vi "View.vi"(8 "error in (no error)":errorcluster, 11 "Worker In":refnum<class "Worker.lvclass">) -> (0 "error out":errorcluster)   [LabVIEW 2020, in "Worker.lvclass"]
doc: "This VI implements the main UI of the process. A reference to this VI should be set using the Set View VI Reference.vi method when the VI is started."
uses:
  Worker.lvclass
  C:/Program Files (x86)/National Instruments/LabVIEW 2020/vi.lib/Astemes/Triarc Framework/Process/Process.lvclass
  C:/Program Files (x86)/National Instruments/LabVIEW 2020/vi.lib/Astemes/Triarc Framework/View/View.lvclass
  <vilib>/Astemes/Triarc Framework/View/View.lvclass/View.ctl
  <vilib>/Astemes/Triarc Framework/View/View.lvclass
  <vilib>/Astemes/Triarc Framework/Process/Process.lvclass
panel:
  out "Name":string
  out "Worker Type":string="Barista"
  out "Orders Filled This Shift":u32
  out "Status":string
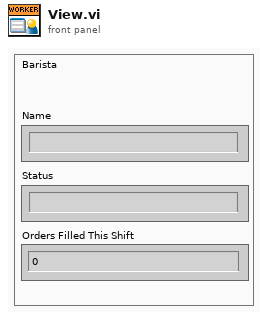
[diagram p1: front panel]
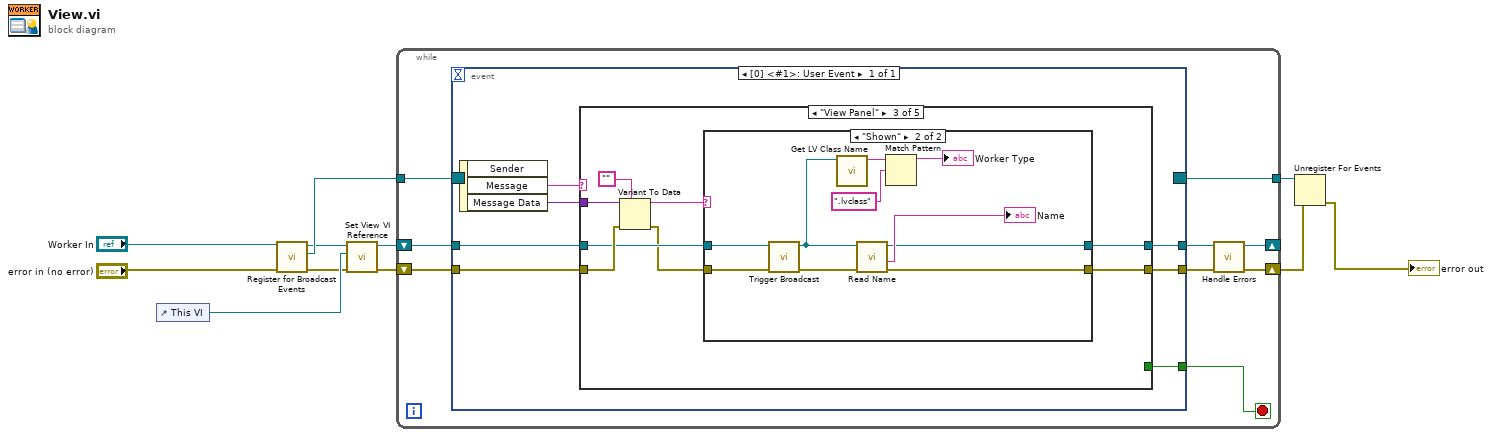
[diagram p0: block diagram]
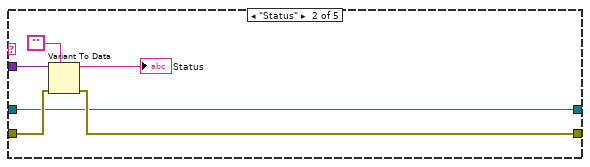
[diagram p3: hidden frame]
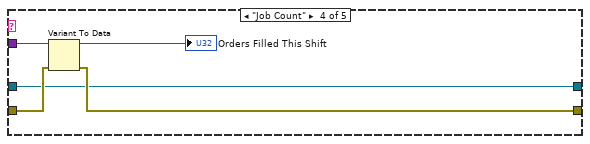
[diagram p5: hidden frame]
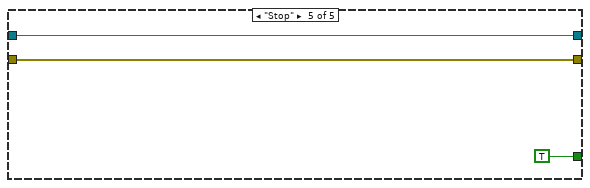
[diagram p6: hidden frame]
diagram:
  n1 = control-ref of="This VI"() -> (w10:refnum<vi>)
  n2 = call <vilib>:"Register for Broadcast Events.vi"("error in (no error)"="error in (no error)", "Process In"="Worker In") -> ("error out"=w8:errorcluster, "Event Registration Refnum Out"=w9:refnum<event-registration>, "Process Out"=w7:refnum<class "Worker.lvclass">)  [unwired: 7 in]
  n3 = call <vilib>:"Set View VI Reference.vi"("error in (no error)"=w8, "View VI Reference"=w10, "View In"=w7) -> ("error out"=w6:errorcluster, "View Out"=w5:refnum<class "Worker.lvclass">)  [unwired: 7 in]
  n4 = while {
    shift-right: [w14] -> _
    shift-left: w5 -> [w20]
    shift-right: [w12] -> w4
    shift-left: w6 -> [w18]
    tunnel: w9 -> [w17]
    tunnel: [w16] -> w3
    stop <- w15 stop-if-true
    n5 = event shown="[0] <#1>: User Event" {
      selector: w17 -> [_]
      dyn-events: [_] -> w16
      timeout: _ -> [_]
      tunnel: w20 -> [w27]
      tunnel: [w26] -> w19
      tunnel: w18 -> [w24]
      tunnel: [w25] -> w13
      tunnel: [w22] -> w15
      event User Event {
        n6 = event-data() -> ("Message"=w23:string, "Message Data"=w21:variant)  [unwired: 1 in, 1 out]
        n7 = case shown="\"View Panel\"" w23 {
          tunnel: w27 -> [w29 w30 w39 w57 w63]
          tunnel: [w29 w30 w38 w57 w63] -> w26
          tunnel: [w28 w31 w36 w58 w62] -> w25
          tunnel: w24 -> [w28 w34 w42 w59 w62]
          tunnel: [_ _ _ _ TRUE] -> w22
          tunnel: w21 -> [_ w35 w43 w60 _]
          frame Default {
          }
          frame "Status" {
            n8 = Variant To Data(error in=w34, type="", Variant=w35) -> (data=→"Status":string, error out=w31:errorcluster)
          }
          frame "View Panel" {
            n9 = Variant To Data(error in=w42, type="", Variant=w43) -> (data=w40:string, error out=w37:errorcluster)
            n10 = case shown="\"Shown\"" w40 {
              tunnel: w39 -> [w45 w47]
              tunnel: [w45 w51] -> w38
              tunnel: w37 -> [w44 w50]
              tunnel: [w44 w49] -> w36
              frame Default {
              }
              frame "Shown" {
                n11 = call <vilib>:"Trigger Broadcast.vi"("error in (no error)"=w50, "Process in"=w47) -> ("error out"=w48:errorcluster, "Process out"=w46:refnum<class "Worker.lvclass">)  [unwired: 8 in]
                n12 = call <vilib>:"Get LV Class Name.vi"("object"=w46) -> ("class name"=w53:string)  [unwired: 9 in, 1 out]
                n13 = call <vilib>:"Read Name.vi"("error in (no error)"=w48, "Process In"=w46) -> ("error out"=w49:errorcluster, "Name"=→"Name":string, "Process Out"=w51:refnum<class "Worker.lvclass">)  [unwired: 6 in, 1 out]
                n14 = Match Pattern(string=w53, regular expression=".lvclass") -> (before substring=→"Worker Type":string)  [unwired: 1 in, 3 out]
              }
            }
          }
          frame "Job Count" {
            n15 = Variant To Data(error in=w59, Variant=w60) -> (data=→"Orders Filled This Shift":u32, error out=w58:errorcluster)  [unwired: 1 in]
          }
          frame "Stop" {
          }
        }
      }
    }
    n16 = call-dynamic "Handle Errors.vi"("error in (no error)"=w13, "Process In"=w19) -> ("error out"=w12:errorcluster, "Process Out"=w14:refnum<class "Worker.lvclass">)  [unwired: 8 in]
  }
  n17 = Unregister For Events(event registration refnum=w3, error in=w4) -> (error out=→"error out":errorcluster)
